vi "Save CSV.vi"(7 "CSV FILE PATH Ref":refnum<vi>, 8 "error in (no error)":errorcluster, 11 "MONITOR TABLE Ref":refnum<vi>) -> (0 "error out":errorcluster)   [LabVIEW 2025, in "I2C Bus Monitor UI.lvlib"]
uses:
  I2C Bus Monitor UI.lvlib
  <vilib>/Utility/file.llb/Write Delimited Spreadsheet (string).vi
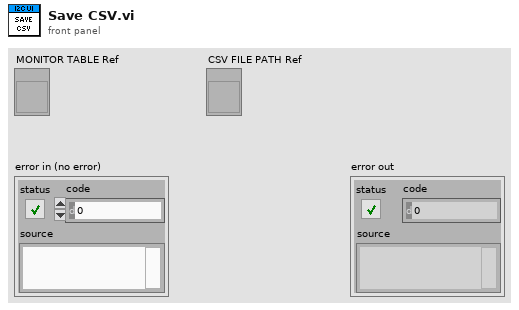
[diagram p1: front panel]
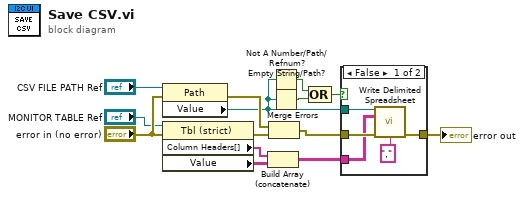
[diagram p0: block diagram]
diagram:
  n1 = property class="Path"(reference="CSV FILE PATH Ref", error in="error in (no error)") -> (error out=w14:errorcluster, "Value"=w1:path)  [unwired: 1 out]
  n2 = property class="Tbl (strict)"(reference="MONITOR TABLE Ref", error in="error in (no error)") -> (error out=w10:errorcluster, "Column Headers[]"=w5:string[], "Value"=w6:string[][])  [unwired: 1 out]
  n3 = Build Array (concatenate)(w5, w6) -> (w7:string[][])
  n4 = Merge Errors(w14, w10) -> (w9:errorcluster)
  n5 = Not A Number/Path/Refnum?(number/path/refnum=w1) -> (NaN/Path/Refnum?=w2:bool)
  n6 = Empty String/Path?(string/path=w1) -> (empty?=w4:bool)
  n7 = Compound Arithmetic op=OR(w2, w4) -> (w3:bool)
  n8 = case shown="False" w3 {
    tunnel: w1 -> [w19 _]
    tunnel: w9 -> [w18 w20]
    tunnel: [w16 w20] -> w8
    tunnel: w7 -> [w15 _]
    frame False {
      n9 = call-poly <vilib>:"Write Delimited Spreadsheet.vi"("file path (dialog if empty)"=w19, "2D data"=w15, "error in (no error)"=w18, "delimiter (\\t)"="," ("delimiter (\\t)")) -> ("error out"=w16:errorcluster)  [unwired: 10 in, 1 out]
    }
    frame True {
    }
  }
  "error out" <- w8
